vi "SetLimit_axis.vi"(6 "max":dbl, 7 "min":dbl, 8 "error in (no error)":errorcluster, 9 "real pos zero":dbl, 10 "Axis":T1 items=["1"=1, "2"=2, "3"=3, "4"=4], 11 "DelayLine in":refnum<class "DelayLine.lvclass">) -> (0 "error out":errorcluster, 3 "DelayLine out":refnum<class "DelayLine.lvclass">)   [LabVIEW 2019, in "DelayLine.lvclass"]
uses:
  DelayLine.lvclass
  DelayLineLS4/LS4 axis.ctl
  DelayLineLS4/LS4_parameters.ctl
  DelayLine.lvclass/DelayLine.ctl
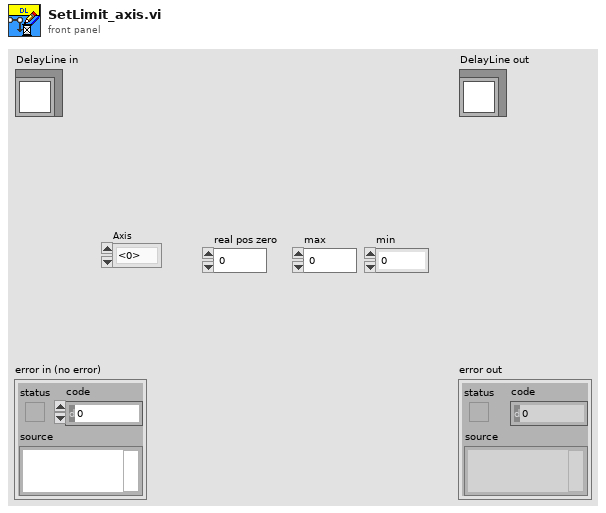
[diagram p1: front panel]
types:
  T1 = typedef "DelayLine.lvclass/LS4 axis.ctl" = u16
  T2 = typedef "DelayLine.lvclass/LS4_parameters.ctl" = string
  T3 = cluster{"X":cluster{"Min":dbl, "Max":dbl}, "Y":cluster{"Min":dbl, "Max":dbl}, "Z":cluster{"Min":dbl, "Max":dbl}, "A":cluster{"Min":dbl, "Max":dbl}}
  T4 = cluster{"Limits[0]":cluster{"Min":dbl, "Max":dbl}, "Limits[1]":cluster{"Min":dbl, "Max":dbl}, "Limits[2]":cluster{"Min":dbl, "Max":dbl}, "Limits[3]":cluster{"Min":dbl, "Max":dbl}, "Limits[4]":cluster{"Min":dbl, "Max":dbl}, "Limits[5]":cluster{"Min":dbl, "Max":dbl}, "Limits[6]":cluster{"Min":dbl, "Max":dbl}, "Limits[7]":cluster{"Min":dbl, "Max":dbl}, "Limits[8]":cluster{"Min":dbl, "Max":dbl}}
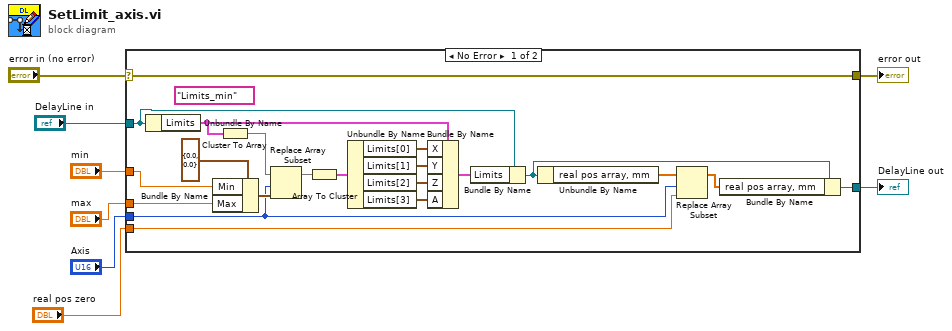
[diagram p0: block diagram]
diagram:
  n1 = case shown="No Error" "error in (no error)" {
    selector: "error in (no error)" -> [w29 w31]
    tunnel: "DelayLine in" -> [w15 w30]
    tunnel: [w14 w30] -> w5
    tunnel: [w29 w31] -> w6
    tunnel: "Axis" -> [w9 _]
    tunnel: "min" -> [w28 _]
    tunnel: "max" -> [w27 _]
    tunnel: "real pos zero" -> [w12 _]
    frame No Error {
      (unwired) T2 "Limits_min" ("Section")
      n2 = Unbundle By Name(w15) -> ("Limits"=w22:T3)
      n3 = Bundle By Name(cluster=cluster{"Min":dbl, "Max":dbl} {"Min"=0.0, "Max"=0.0} ("element"), "Min"=w28, "Max"=w27) -> (w25:cluster{"Min":dbl, "Max":dbl})
      n4 = Cluster To Array(cluster=w22) -> (array=w24:cluster{"Min":dbl, "Max":dbl}[])
      n5 = Replace Array Subset(array=w24, new element=w25, index=w9) -> (w23:cluster{"Min":dbl, "Max":dbl}[])
      n6 = Array To Cluster(array=w23) -> (cluster=w21:T4)
      n7 = Unbundle By Name(w21) -> ("Limits[0]"=w20:cluster{"Min":dbl, "Max":dbl}, "Limits[1]"=w19:cluster{"Min":dbl, "Max":dbl}, "Limits[2]"=w18:cluster{"Min":dbl, "Max":dbl}, "Limits[3]"=w17:cluster{"Min":dbl, "Max":dbl})
      n8 = Bundle By Name(cluster=w22, "X"=w20, "Y"=w19, "Z"=w18, "A"=w17) -> (w16:T3)
      n9 = Bundle By Name(cluster=w15, "Limits"=w16) -> (w10:refnum<class "DelayLine.lvclass">)
      n10 = Unbundle By Name(w10) -> ("real pos array, mm"=w13:dbl[])
      n11 = Replace Array Subset(array=w13, new element=w12, index=w9) -> (w11:dbl[])
      n12 = Bundle By Name(cluster=w10, "real pos array, mm"=w11) -> (w14:refnum<class "DelayLine.lvclass">)
    }
    frame Error {
    }
  }
  "error out" <- w6
  "DelayLine out" <- w5
